vi "DriveTest.vi"() -> ()   [LabVIEW 2009]
doc: "This is a test VI for robot driving"
uses:
  Drive.lvlib
  Motor.lvlib
  FPGA.lvlib
  Servo.lvlib
panel:
  in  "stop 2":bool
  in  "Speed limit":dbl
  in  "Right_Distance":dbl
  in  "Left_Distance":dbl
  in  "Y_Speed":dbl(slide) min=-1.0 max=1.0 scale=-1.0..1.0
  in  "X_Speed":dbl(slide) min=-1.0 max=1.0 scale=-1.0..1.0
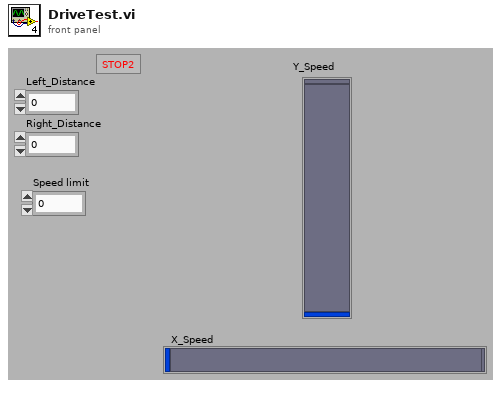
[diagram p1: front panel]
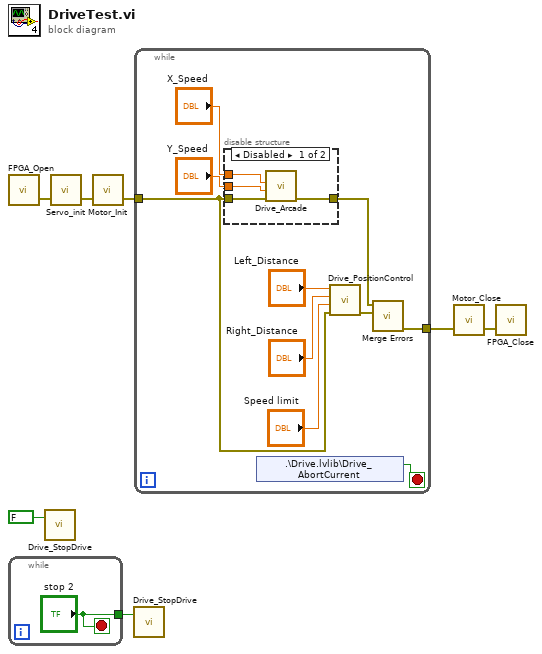
[diagram p0: block diagram]
diagram:
  n1 = call "FPGA_Open.vi"() -> ("error out"=w1:errorcluster)  [unwired: 3 in]
  n2 = while {
    tunnel: ["stop 2"] -> w4
    stop <- "stop 2" stop-if-true
  }
  n3 = call "Drive_StopDrive.vi"("Abort?"=FALSE) -> ()  [unwired: 2 in, 1 out]
  n4 = call "Servo_init.vi"("error in (no error)"=w1) -> ("error out"=w2:errorcluster)  [unwired: 2 in]
  n5 = call "Motor_Init.vi"("error in"=w2) -> ("error out"=w7:errorcluster)  [unwired: 2 in]
  n6 = call "Drive_StopDrive.vi"("Abort?"=w4) -> ()  [unwired: 2 in, 1 out]
  n7 = while {
    tunnel: [w15] -> w6
    tunnel: w7 -> [w13]
    stop <- w9 stop-if-true
    n8 = disable-structure shown="Disabled" {
      disable-tunnel: "X_Speed" -> [w22 _]
      disable-tunnel: "Y_Speed" -> [w21 _]
      disable-tunnel: [w20 _] -> w16
      disable-tunnel: w13 -> [w19 _]
      frame #0 {
        n9 = call "Drive_Arcade.vi"("error in"=w19, "Y_Speed"=w21, "X_Speed"=w22) -> ("error out"=w20:errorcluster)  [unwired: 8 in]
      }
      frame #1 {
      }
    }
    n10 = shared-variable ".\\Drive.lvlib\\Drive_AbortCurrent"() -> (w9:bool)  [unwired: 1 in, 1 out]
    n11 = call "Drive_PositionControl.vi"("error in"=w13, "Speed limit"="Speed limit", "Right_Distance"="Right_Distance", "Left_Distance"="Left_Distance") -> ("error out"=w14:errorcluster)  [unwired: 7 in]
    n12 = call <vilib>:"Merge Errors.vi"("error in 2 (no error)"=w14, "error in 1 (no error)"=w16) -> ("error out"=w15:errorcluster)  [unwired: 5 in]
  }
  n13 = call "Motor_Close.vi"("error in"=w6) -> ("error out"=w5:errorcluster)  [unwired: 2 in]
  n14 = call "FPGA_Close.vi"("error in (no error)"=w5) -> ()  [unwired: 2 in, 1 out]
